vi "PLC.Dial750.vi"(7 "PLC Indicator":refnum<vi>, 8 "Is Child":bool, 9 "Config Dir":path=path "C:/MTE/Circle Test/Config", 10 "Name":string="PLC", 11 "TE Q":refnum<queue>) -> ()   [LabVIEW 2018]
uses:
  Controls/PLC.750 Variables.ctl
  <vilib>/KATE/Queues/Q.Element.ctl
  Controls/PLC750.Connection Config.ctl
  Controls/PLC750.Variable Names.ctl
  <vilib>/KATE/Queues/Queue Utils.lvlib
  <instrlib>/_Ackermann Automation/TwinCAT ADS Library/TcAdsLV_TCP/TcAdsLV_TCP_3.lvlib
  <vilib>/KATE/Scheduler/Scheduler.lvlib
  <vilib>/KATE/Time/Time Utils.lvlib
panel:
  out "Test State 2":T1(radio)
  out "Connected":bool
  in  "Tab Control":enum32{"Operate", "Config"}(tab)
  in  "Enabled":bool=TRUE
  in  "Clear Start":bool
  in  "Seq Done FAIL":bool
  in  "Clear Done":bool
  in  "Clear Pass":bool
  in  "Set Running":bool
  in  "Seq Run":bool
  in  "Seq Done PASS":bool
  in  "Seq Start Capture":bool
  out "Status":string
  out "Nest":string
  out "SN":string
  out "Test State":T1(radio)
  out "Reading":bool
  out "PLC Variables":T2
  in  "Set Ready":bool
  out "Test Running":bool
  out "Result":string="PASS"
  out "Read Time":timestamp format="%<%.3X>T"
  in  "PLC Read Interval(s)":dbl=0.1 caption="Read Interval(s)" format="%#_13g"
  in  "Read Data":bool
  in  "Clear Running":bool
  in  "Exit":bool
  in  "Clear Error":bool
  out "Error Time":timestamp format="%<%.3X>T"
  out "Connection Info":T3={"Net ID Target"="5.49.203.74.1.1", "Net ID Source"="192.168.1.18.1.1", "IP Address Target"="172.16.113.5", "Target Port"=851}
  out "Error":errorcluster
  in  "Retry Sec":dbl=2.0 caption="Connect Retry Sec" format="%#_13g"
  out "VarNames":T4={"SN"="g.SN", "Nest"="g.Nest", "Ready"="g.Ready", "Start"="g.Start", "Pass"="g.Pass", "Done"="g.Done", "Running"="GVL.gDone"}
  in  "Reset":bool
  in  "Single Step":bool
  in  "Emulate":bool
  out "Activation Ok":bool
  # "PLC Connection Manager"
  # "*** Sequence ***\nPLC -> \n  Set Done=F\n  Set Pass=F\n  Set Start=F\n  Set Running=F\n  Set Nest = Value\n  Set SN = Value\n  Set Ready=T\n\nTE -> \n  Get Nest\n  Get SN\n  Set Ready=F\n  Launch Test Sequence\n  \nTE -> \n  Test ready for tracked objects to spin\n   Set Start=T\n\nPLC -> \n  Set Running=T\n  Spin objects 360 deg\n  Set Running=F\n\nTE -> \n  Continue test\n  Test Complete\n   Set Pass = Value (T = Pass, F = Fail or Error)\n   Set Done=T\n\nPLC -> \n   Set Done=F"
  # "Simulate PLC"
  # "Test Executive Data"
  # "Simulate TE"
  # "Set Start"
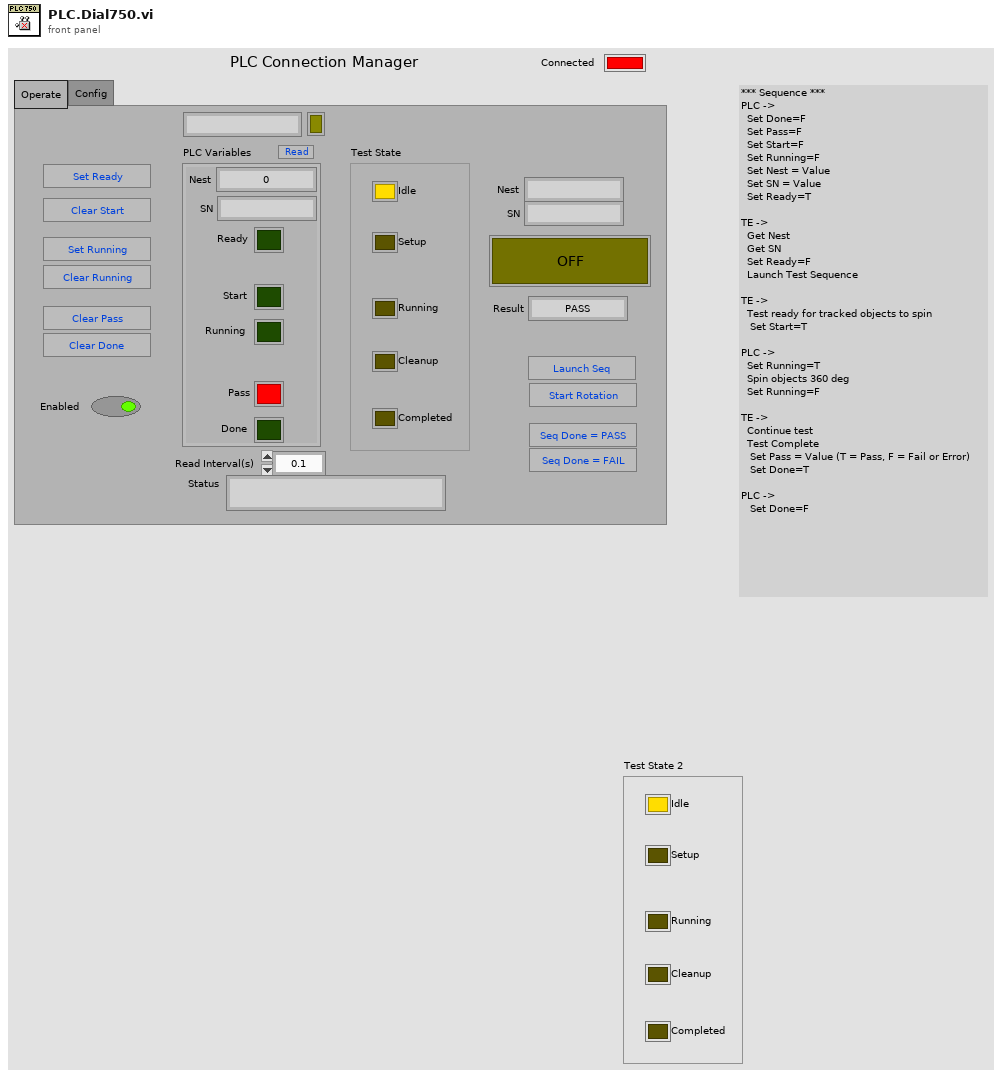
[diagram p1: front panel]
types:
  T1 = enum32{"Idle", "Setup", "Running", "Cleanup", "Completed"}
  T2 = typedef "PLC.750 Variables.ctl" = cluster{"Nest":i32, "SN":string, "Ready":bool, "Start":bool, "Pass":bool, "Done":bool, "Running":bool}
  T3 = typedef "PLC750.Connection Config.ctl" = cluster{"Net ID Target":string, "Net ID Source":string, "IP Address Target":string, "Target Port":u16}
  T4 = typedef "PLC750.Variable Names.ctl" = cluster{"SN":string, "Nest":string, "Ready":string, "Start":string, "Pass":string, "Done":string, "Running":string}
  T5 = enum8{"Enabled", "Disabled", "Disabled and Grayed Out"}
  T6 = enum32{"invalid app kind", "Development System", "Run Time System", "Student Edition", "Embedded LabVIEW", "Evaluation", "Custom"}
  T7 = enum32{"Invalid", "Standard", "Closed", "Hidden", "Minimized", "Maximized"}
  T8 = cluster{"VarConfig":T4, "Var Names":string[][], "Data":T2, "Session Ref":u32, "Connected":bool, "ConCfg":T3, "State":enum32{"Idle", "Setup", "Running", "Cleanup", "Completed"}, "PLC Indicator":refnum<vi>}
  T9 = typedef "TcAdsLV_Common_3.lvlib/ClusterAdsSymbolEntry.ctl" = cluster{"Index Group":u32, "Index Offset":u32, "Size":u32, "Data Type":u32, "Flags":u32, "Name":string, "Type":string, "Comment":string}
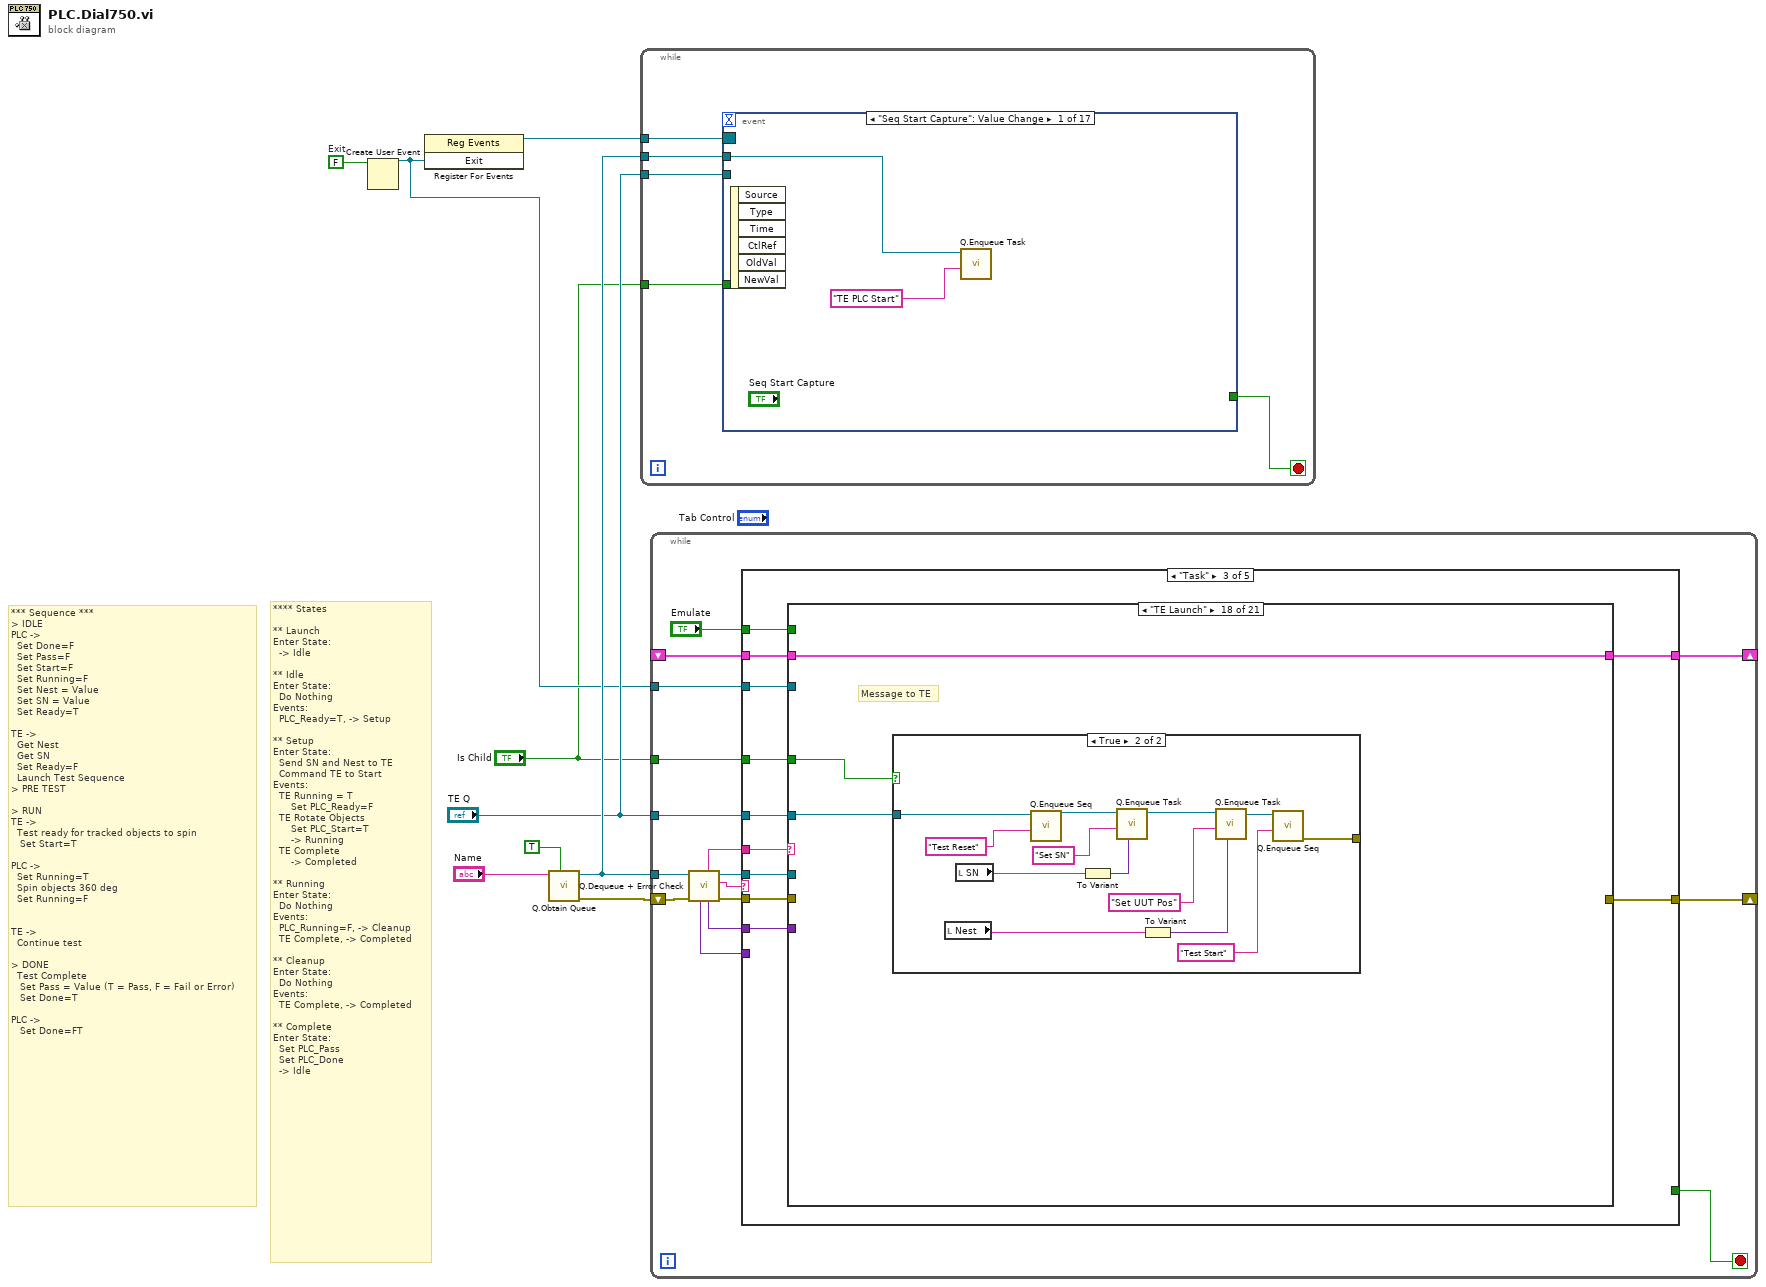
[diagram p0: block diagram]
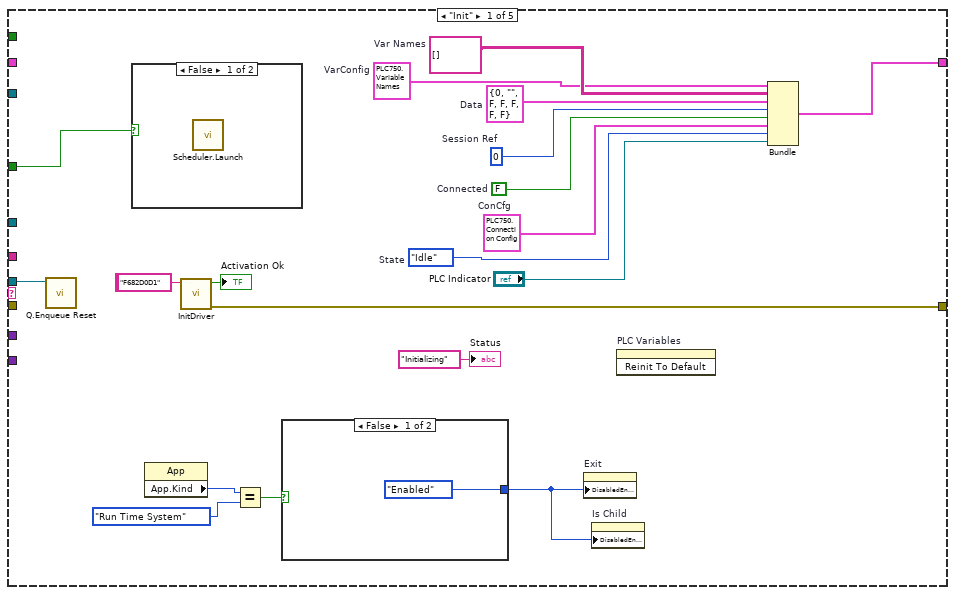
[diagram p2: hidden frame]
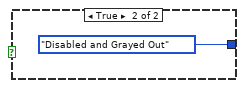
[diagram p3: hidden frame]
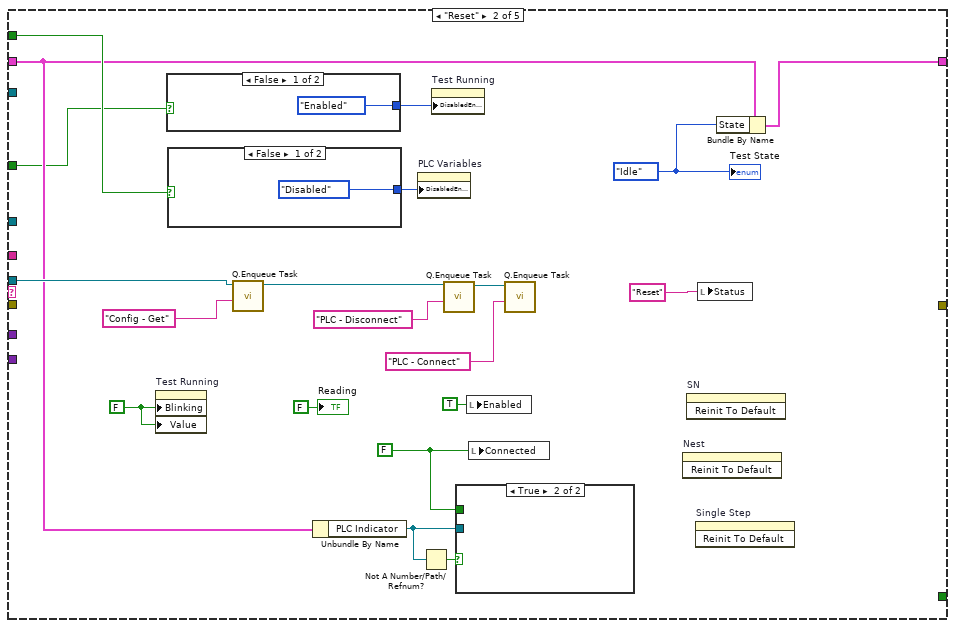
[diagram p5: hidden frame]
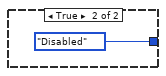
[diagram p6: hidden frame]
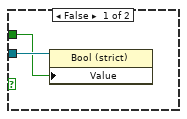
[diagram p7: hidden frame]
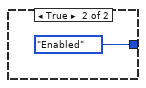
[diagram p8: hidden frame]
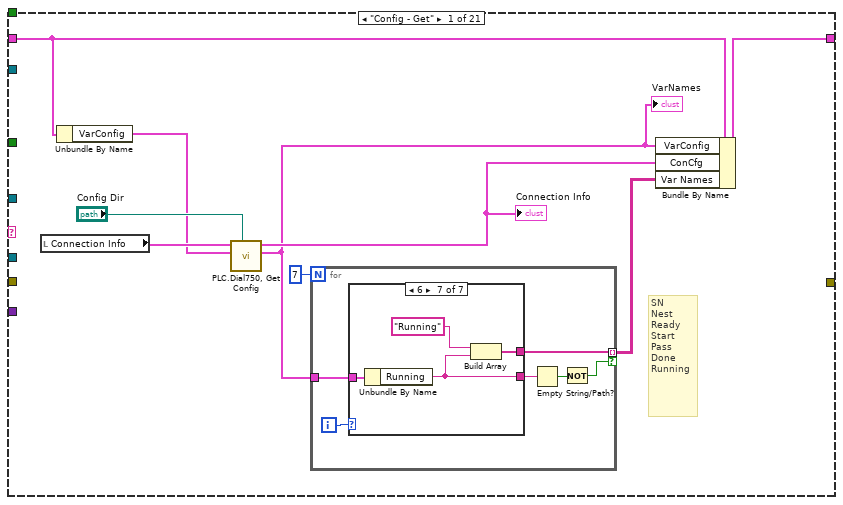
[diagram p9: hidden frame]
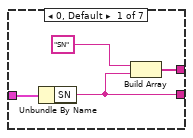
[diagram p10: hidden frame]
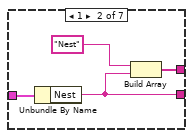
[diagram p11: hidden frame]
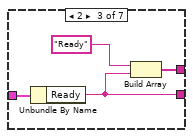
[diagram p12: hidden frame]
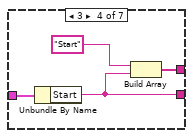
[diagram p13: hidden frame]
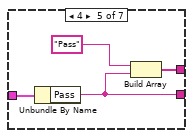
[diagram p14: hidden frame]
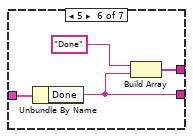
[diagram p15: hidden frame]
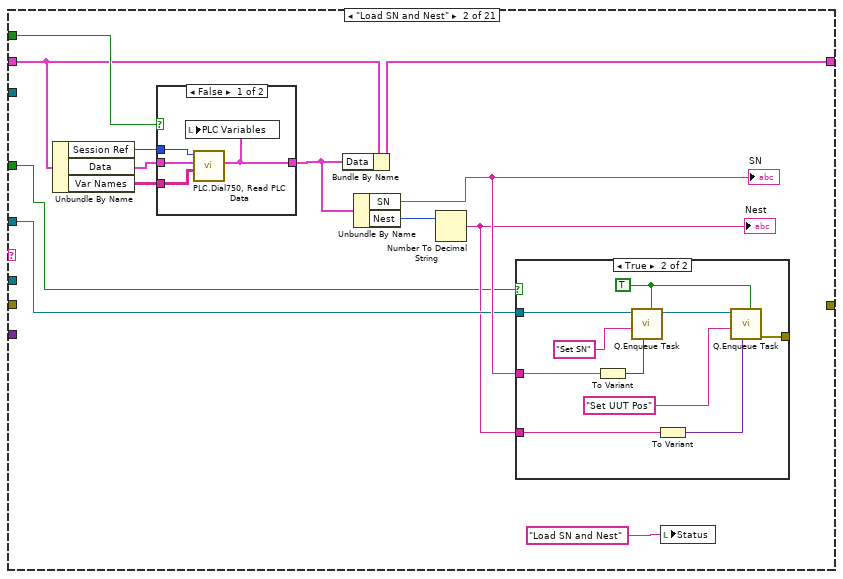
[diagram p16: hidden frame]
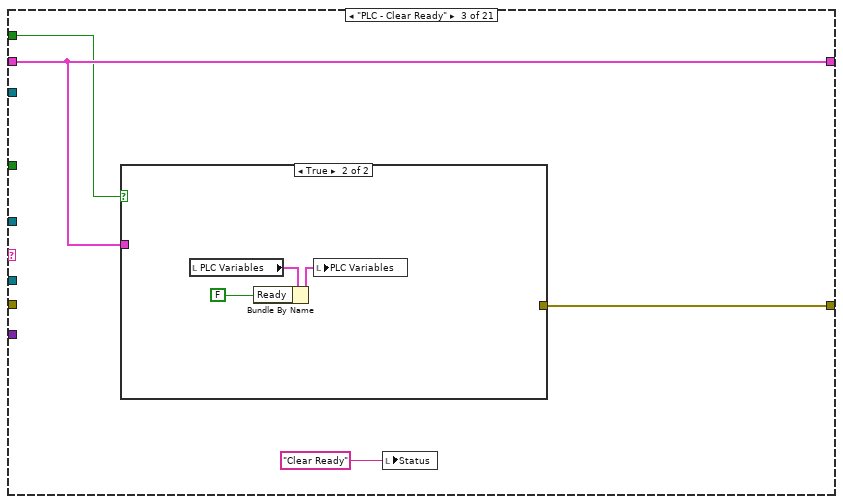
[diagram p19: hidden frame]
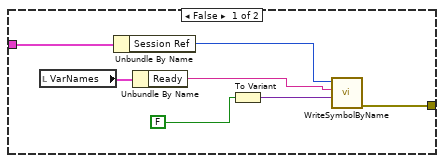
[diagram p20: hidden frame]
diagram:
  w6 = FALSE  # Exit
  # "**** States\n\n** Launch\nEnter State: \n  -> Idle\n\n** Idle\nEnter State: \n  Do Nothing\nEvents:\n  PLC_Ready=T, -> Setup\n\n** Setup\nEnter State: \n  Send SN and Nest to TE\n  Command TE to Start\nEvents:\n  TE Running = T\n      Set PLC_Ready=F\n  TE Rotate Objects\n      Set PLC_Start=T\n      -> Running\n  TE Complete\n      -> Completed\n\n** Running\nEnter State: \n  Do Nothing\nEvents:\n  PLC_Running=F, -> Cleanup\n  TE Complete, -> Completed\n\n** Cleanup\nEnter State: \n  Do Nothing\nEvents:\n  TE Complete, -> Completed\n\n** Complete\nEnter State: \n  Set PLC_Pass\n  Set PLC_Done \n  -> Idle"
  # "*** Sequence ***\n> IDLE\nPLC -> \n  Set Done=F\n  Set Pass=F\n  Set Start=F\n  Set Running=F\n  Set Nest = Value\n  Set SN = Value\n  Set Ready=T\n\nTE -> \n  Get Nest\n  Get SN\n  Set Ready=F\n  Launch Test Sequence\n> PRE TEST\n  \n> RUN\nTE -> \n  Test ready for tracked objects to spin\n   Set Start=T\n\nPLC -> \n  Set Running=T\n  Spin objects 360 deg\n  Set Running=F\n\n\nTE -> \n  Continue test\n\n> DONE\n  Test Complete\n   Set Pass = Value (T = Pass, F = Fail or Error)\n   Set Done=T\n\nPLC -> \n   Set Done=FT"
  n1 = Create User Event(user event datatype=w6) -> (user event=w2:refnum<user-event>)  [unwired: 1 in, 1 out]
  n2 = register-events(w2) -> (reference out=w5:refnum<event-registration>)  [unwired: 2 in, 1 out]
  n3 = call <vilib>:"Q.Obtain Queue.vi"("Enqueue Init"=TRUE, "Q Name"="Name") -> ("error out"=w3:errorcluster, "Q Out"=w7:refnum<queue>)  [unwired: 7 in, 1 out]
  n4 = while {
    tunnel: w7 -> [w14]
    tunnel: w5 -> [w13]
    tunnel: "TE Q" -> [w12]
    tunnel: "Is Child" -> [w10]
    stop <- w11 stop-if-true
    n5 = event shown="[0] \"Seq Start Capture\": Value Change" {
      selector: w13 -> [_ _ _ _ _ _ _ _ _ _ _ _ _ _ _ _ _]
      dyn-events: _ -> [_ _ _ _ _ _ _ _ _ _ _ _ _ _ _ _ _]
      timeout: _ -> [_ _ _ _ _ _ _ _ _ _ _ _ _ _ _ _ _]
      tunnel: w14 -> [w16 _ _ w21 w22 _ w32 w38 _ _ _ _ _ _ w57 w63 w64]
      tunnel: w12 -> [_ _ _ _ _ _ _ _ _ _ _ _ _ _ _ _ _]
      tunnel: [_ _ _ _ _ _ _ _ TRUE _ _ _ _ _ w56 TRUE _] -> w11
      tunnel: w10 -> [_ _ _ _ _ _ _ _ _ _ _ _ _ _ w55 _ _]
      event "Seq Start Capture": Value Change {
        n6 = event-data() -> ()  [unwired: 1 in, 6 out]
        n7 = call <vilib>:"Q.Enqueue Task.vi"("Task Name"="TE PLC Start", "Q In"=w16) -> ()  [unwired: 8 in, 2 out]
      }
      event "Emulate": Value Change {
        n8 = event-data() -> ("NewVal"=w17:bool)  [unwired: 1 in, 5 out]
        n9 = case shown="False" w17 {
          tunnel: [T5."Disabled" ("Disabled") T5."Enabled" ("Disabled")] -> w18
          frame False {
          }
          frame True {
          }
        }
        n10 = property on="PLC Variables" class="Clust (strict)"("DisabledEnum"=w18) -> ()  [unwired: 2 in, 2 out]
      }
      event "Clear Error": Value Change {
        n11 = event-data() -> ()  [unwired: 1 in, 6 out]
        n12 = invoke on="Error" class="Clust (strict)" method="Reinit To Default"() -> ()  [unwired: 3 in, 3 out]
      }
      event "Reset": Value Change {
        n13 = event-data() -> ()  [unwired: 1 in, 6 out]
        n14 = call <vilib>:"Q.Enqueue Reset.vi"("Q In"=w21) -> ()  [unwired: 9 in, 2 out]
      }
      event "Read Data": Value Change {
        n15 = event-data() -> ()  [unwired: 1 in, 6 out]
        n16 = call <vilib>:"Q.Enqueue Task.vi"("Task Name"="PLC - Read Data", "Q In"=w22) -> ()  [unwired: 8 in, 2 out]
      }
      event "Set Ready": Value Change {
        n17 = event-data() -> ()  [unwired: 1 in, 6 out]
        n18 = local read "PLC Variables"() -> (w25:T2)
        n19 = Bundle By Name(cluster=w25, "Ready"=TRUE) -> (w26:T2)
        n20 = local write "PLC Variables"(w26) -> ()
      }
      event "Seq Done PASS": Value Change {
        n21 = event-data() -> ()  [unwired: 1 in, 6 out]
        n22 = To Variant(anything="PASS") -> (Variant=w27:variant)
        n23 = call <vilib>:"Q.Enqueue Task.vi"("Data1"=w27, "Task Name"="TE Result", "Q In"=w32) -> ("Q Out"=w30:refnum<queue>)  [unwired: 7 in, 1 out]
        n24 = call <vilib>:"Q.Enqueue Task.vi"("Task Name"="TE Complete", "Q In"=w30) -> ()  [unwired: 8 in, 2 out]
      }
      event "Seq Done FAIL": Value Change {
        n25 = event-data() -> ()  [unwired: 1 in, 6 out]
        n26 = To Variant(anything="FAIL") -> (Variant=w33:variant)
        n27 = call <vilib>:"Q.Enqueue Task.vi"("Data1"=w33, "Task Name"="TE Result", "Q In"=w38) -> ("Q Out"=w36:refnum<queue>)  [unwired: 7 in, 1 out]
        n28 = call <vilib>:"Q.Enqueue Task.vi"("Task Name"="TE Complete", "Q In"=w36) -> ()  [unwired: 8 in, 2 out]
      }
      event User Event {
        n29 = event-data() -> ()  [unwired: 1 in, 4 out]
      }
      event "Set Running": Value Change {
        n30 = event-data() -> ()  [unwired: 1 in, 6 out]
        n31 = local read "PLC Variables"() -> (w40:T2)
        n32 = Bundle By Name(cluster=w40, "Running"=TRUE ("Ready")) -> (w41:T2)
        n33 = local write "PLC Variables"(w41) -> ()
      }
      event "Clear Done": Value Change {
        n34 = event-data() -> ()  [unwired: 1 in, 6 out]
        n35 = local read "PLC Variables"() -> (w43:T2)
        n36 = Bundle By Name(cluster=w43, "Done"=FALSE ("Ready")) -> (w44:T2)
        n37 = local write "PLC Variables"(w44) -> ()
      }
      event "Clear Start": Value Change {
        n38 = event-data() -> ()  [unwired: 1 in, 6 out]
        n39 = local read "PLC Variables"() -> (w46:T2)
        n40 = Bundle By Name(cluster=w46, "Start"=FALSE ("Ready")) -> (w47:T2)
        n41 = local write "PLC Variables"(w47) -> ()
      }
      event "Clear Pass": Value Change {
        n42 = event-data() -> ()  [unwired: 1 in, 6 out]
        n43 = local read "PLC Variables"() -> (w49:T2)
        n44 = Bundle By Name(cluster=w49, "Pass"=FALSE ("Ready")) -> (w50:T2)
        n45 = local write "PLC Variables"(w50) -> ()
      }
      event "Clear Running": Value Change {
        n46 = event-data() -> ()  [unwired: 1 in, 6 out]
        n47 = local read "PLC Variables"() -> (w52:T2)
        n48 = Bundle By Name(cluster=w52, "Running"=FALSE ("Ready")) -> (w53:T2)
        n49 = local write "PLC Variables"(w53) -> ()
      }
      event Panel Close? {
        n50 = event-data() -> ()  [unwired: 1 in, 4 out]
        n51 = case shown="False" w55 {
          tunnel: w57 -> [w60 _]
          tunnel: [TRUE _] -> w56
          frame False {
            n52 = call <vilib>:"Q.Enqueue Exit.vi"("Q In"=w60) -> ()  [unwired: 9 in, 2 out]
          }
          frame True {
            n53 = control-ref of="This VI"() -> (w61:refnum<vi>)
            n54 = invoke class="VI" method="FP.Close"(reference=w61) -> ()  [unwired: 2 in, 3 out]
          }
        }
        n55 = event-data("Discard?"=TRUE) -> ()  [unwired: 1 in, 1 out]
      }
      event "Exit": Value Change {
        n56 = event-data() -> ()  [unwired: 1 in, 6 out]
        n57 = call <vilib>:"Q.Enqueue Exit.vi"("Q In"=w63) -> ()  [unwired: 9 in, 2 out]
      }
      event "Seq Run": Value Change {
        n58 = event-data() -> ()  [unwired: 1 in, 6 out]
        n59 = call <vilib>:"Q.Enqueue Task.vi"("Task Name"="TE Running", "Q In"=w64) -> ()  [unwired: 8 in, 2 out]
      }
    }
  }
  n60 = while {
    tunnel: w7 -> [w81]
    shift-right: [w73] -> _
    shift-left: _ -> [w80]
    tunnel: "TE Q" -> [w71]
    shift-right: [w69] -> _
    shift-left: w3 -> [w70]
    tunnel: w2 -> [w68]
    tunnel: "Is Child" -> [w66]
    stop <- w72 stop-if-true
    n61 = call <vilib>:"Q.Dequeue + Error Check.vi"("Error In"=w70, "Q In"=w81) -> ("error out"=w77:errorcluster, "Cmd"=w79:string, "Q Out"=w78:refnum<queue>, "Data1"=w75:variant, "Sub"=w76:string, "Data2"=w74:variant)  [unwired: 4 in]
    n62 = case shown="\"Task\"" w79 {
      tunnel: w80 -> [_ w106 w135 w481 w495]
      tunnel: w78 -> [w93 w116 w137 _ _]
      tunnel: w77 -> [_ _ w136 w484 _]
      tunnel: w76 -> [_ _ w139 w485 _]
      tunnel: w75 -> [_ _ w138 w482 _]
      tunnel: w74 -> [_ _ _ _ _]
      tunnel: [w100 w117 w134 w481 w495] -> w73
      tunnel: [_ _ _ _ TRUE] -> w72
      tunnel: w71 -> [_ _ w130 _ _]
      tunnel: [w97 _ w133 _ _] -> w69
      tunnel: w68 -> [_ _ w132 _ w494]
      tunnel: "Emulate" -> [_ w112 w131 _ _]
      tunnel: w66 -> [w87 w104 w129 _ w492]
      frame "Init" {
        w90 = T1."Idle"  # State
        w91 = T4 {"SN"="g.SN", "Nest"="g.Nest", "Ready"="g.Ready", "Start"="", "Pass"="g.Pass", "Done"="g.Done", "Running"=""}  # VarConfig
        w92 = string[][] []  # Var Names
        w94 = T3 {"Net ID Target"="5.49.203.74.1.1", "Net ID Source"="192.168.1.18.1.1", "IP Address Target"="172.16.113.5", "Target Port"=851}  # ConCfg
        w95 = FALSE  # Connected
        w96 = u32 0  # Session Ref
        (unwired) "" ("License Number")
        w99 = T2 {"Nest"=0, "SN"="", "Ready"=FALSE, "Start"=FALSE, "Pass"=FALSE, "Done"=FALSE, "Running"=FALSE}  # Data
        n63 = call <vilib>:"Q.Enqueue Reset.vi"("Q In"=w93) -> ()  [unwired: 9 in, 2 out]
        n64 = case shown="False" w87 {
          frame False {
            n65 = call <vilib>:"Scheduler.Launch.vi"() -> ()  [unwired: 9 in, 3 out]
          }
          frame True {
          }
        }
        n66 = property class="App"() -> ("App.Kind"=w85:T6)  [unwired: 2 in, 2 out]
        n67 = call <instrlib>:"InitDriver.vi"("License Number"="F682D0D1") -> ("error out"=w97:errorcluster, "Activation Ok"=→"Activation Ok":bool)  [unwired: 8 in, 1 out]
        n68 = Equal?(x=w85, y=T6."Run Time System" ("Application:Kind")) -> (x = y?=w83:bool)
        n69 = case shown="False" w83 {
          tunnel: [T5."Enabled" ("Disabled") T5."Disabled and Grayed Out" ("Disabled")] -> w86
          frame False {
          }
          frame True {
          }
        }
        n70 = property on="Exit" class="Bool"("DisabledEnum"=w86) -> ()  [unwired: 2 in, 2 out]
        n71 = property on="Is Child" class="Bool (strict)"("DisabledEnum"=w86) -> ()  [unwired: 2 in, 2 out]
        n72 = invoke on="PLC Variables" class="Clust (strict)" method="Reinit To Default"() -> ()  [unwired: 3 in, 3 out]
        n73 = Bundle("VarConfig"=w91, "Var Names"=w92, "Data"=w99, "Session Ref"=w96, "Connected"=w95, "ConCfg"=w94, "State"=w90, "PLC Indicator"="PLC Indicator") -> (w100:T8)  [unwired: 1 in]
        "Status" <- "Initializing" ("Activity")
      }
      frame "Reset" {
        w113 = T1."Idle" ("Test State")
        w107 = FALSE ("Connected")
        w115 = FALSE ("Blinking")
        n74 = property on="Test Running" class="Bool (strict)"("Blinking"=w115, "Value"=w115) -> ()  [unwired: 2 in, 2 out]
        n75 = case shown="False" w104 {
          tunnel: [T5."Enabled" ("Disabled") T5."Disabled" ("Disabled")] -> w105
          frame False {
          }
          frame True {
          }
        }
        n76 = case shown="False" w112 {
          tunnel: [T5."Disabled" ("Disabled") T5."Enabled" ("Disabled")] -> w111
          frame False {
          }
          frame True {
          }
        }
        n77 = call <vilib>:"Q.Enqueue Task.vi"("Task Name"="Config - Get", "Q In"=w116) -> ("Q Out"=w118:refnum<queue>)  [unwired: 8 in, 1 out]
        n78 = Unbundle By Name(w106) -> ("PLC Indicator"=w108:refnum<vi>)
        n79 = property on="PLC Variables" class="Clust (strict)"("DisabledEnum"=w111) -> ()  [unwired: 2 in, 2 out]
        n80 = Not A Number/Path/Refnum?(number/path/refnum=w108) -> (NaN/Path/Refnum?=w109:bool)
        n81 = property on="Test Running" class="Bool (strict)"("DisabledEnum"=w105) -> ()  [unwired: 2 in, 2 out]
        n82 = call <vilib>:"Q.Enqueue Task.vi"("Task Name"="PLC - Disconnect", "Q In"=w118) -> ("Q Out"=w121:refnum<queue>)  [unwired: 8 in, 1 out]
        n83 = case shown="True" w109 {
          tunnel: w108 -> [w126 _]
          tunnel: w107 -> [w125 _]
          frame False {
            n84 = property class="Bool (strict)"(reference=w126, "Value"=w125) -> ()  [unwired: 1 in, 2 out]
          }
          frame True {
          }
        }
        n85 = local write "Enabled"(TRUE ("Enabled")) -> ()
        n86 = local write "Connected"(w107) -> ()
        n87 = call <vilib>:"Q.Enqueue Task.vi"("Task Name"="PLC - Connect", "Q In"=w121) -> ()  [unwired: 8 in, 2 out]
        n88 = invoke on="Nest" class="Str" method="Reinit To Default"() -> ()  [unwired: 3 in, 3 out]
        n89 = invoke on="SN" class="Str" method="Reinit To Default"() -> ()  [unwired: 3 in, 3 out]
        n90 = invoke on="Single Step" class="Bool (strict)" method="Reinit To Default"() -> ()  [unwired: 3 in, 3 out]
        n91 = local write "Status"("Reset" ("Activity")) -> ()
        n92 = Bundle By Name(cluster=w106, "State"=w113) -> (w117:T8)
        "Reading" <- FALSE ("Reading")
        "Test State" <- w113
      }
      frame "Task" {
        n93 = case shown="\"TE Launch\"" w139 {
          tunnel: w138 -> [_ _ _ _ _ _ _ _ _ _ _ _ _ _ w446 _ _ _ w472 _ _]
          tunnel: w137 -> [_ _ _ w233 _ w293 _ _ _ _ w373 w380 _ w438 _ _ w450 _ w469 w475 _]
          tunnel: w136 -> [_ _ _ _ _ w285 _ _ _ _ _ _ _ _ _ _ _ _ _ _ _]
          tunnel: w135 -> [w142 w183 w213 w229 w270 w292 w318 w334 w351 w365 w372 w379 w437 w442 w447 w448 w449 w454 w473 w478 w479]
          tunnel: [w147 w186 w213 w234 w270 w291 w318 w334 w351 w365 w371 w378 w437 w441 w447 w448 w449 w454 w473 w478 w479] -> w134
          tunnel: [_ _ w214 w232 _ w286 w319 w337 w352 _ _ _ _ _ _ _ _ _ _ _ _] -> w133
          tunnel: w132 -> [_ _ _ _ _ _ _ _ _ _ _ _ _ _ _ _ _ _ _ _ _]
          tunnel: w131 -> [_ w184 w212 w230 w273 w281 w316 w333 w350 _ _ _ _ _ _ _ _ _ _ _ _]
          tunnel: w130 -> [_ w192 _ _ _ _ _ _ _ _ _ w377 _ _ _ _ _ w453 _ _ _]
          tunnel: w129 -> [_ w190 _ _ _ _ _ _ _ _ _ _ _ _ _ _ _ w452 _ _ _]
          frame "Config - Get" {
            # "SN\nNest\nReady\nStart\nPass\nDone\nRunning"
            n94 = local read "Connection Info"() -> (w145:T3)
            n95 = Unbundle By Name(w142) -> ("VarConfig"=w141:T4)
            n96 = call "PLC.Dial750, Get Config.vi"("Config Folder"="Config Dir", "VarNames In"=w141, "Connection Info In"=w145) -> ("VarNames"=w143:T4, "Connection Info"=w146:T3)  [unwired: 6 in, 1 out]
            "VarNames" <- w143
            "Connection Info" <- w146
            n97 = for {
              N: 7 -> [_]
              tunnel: w143 -> [w154]
              tunnel: [w152] -> w144 mode=indexing if=w150
              i -> [w153]
              n98 = case shown="6" w153 {
                tunnel: w154 -> [w158 w162 w166 w170 w174 w178 w182]
                tunnel: [w156 w160 w164 w168 w172 w176 w180] -> w152
                tunnel: [w155 w159 w163 w167 w171 w175 w179] -> w149
                frame 0, Default {
                  n99 = Unbundle By Name(w158) -> ("SN"=w155:string)
                  n100 = Build Array("SN", w155) -> (w156:string[])
                }
                frame 1 {
                  n101 = Unbundle By Name(w162) -> ("Nest"=w159:string)
                  n102 = Build Array("Nest", w159) -> (w160:string[])
                }
                frame 2 {
                  n103 = Unbundle By Name(w166) -> ("Ready"=w163:string)
                  n104 = Build Array("Ready", w163) -> (w164:string[])
                }
                frame 3 {
                  n105 = Unbundle By Name(w170) -> ("Start"=w167:string)
                  n106 = Build Array("Start", w167) -> (w168:string[])
                }
                frame 4 {
                  n107 = Unbundle By Name(w174) -> ("Pass"=w171:string)
                  n108 = Build Array("Pass", w171) -> (w172:string[])
                }
                frame 5 {
                  n109 = Unbundle By Name(w178) -> ("Done"=w175:string)
                  n110 = Build Array("Done", w175) -> (w176:string[])
                }
                frame 6 {
                  n111 = Unbundle By Name(w182) -> ("Running"=w179:string)
                  n112 = Build Array("Running", w179) -> (w180:string[])
                }
              }
              n113 = Empty String/Path?(string/path=w149) -> (empty?=w151:bool)
              n114 = Not(x=w151) -> (.not. x?=w150:bool)
            }
            n115 = Bundle By Name(cluster=w142, "VarConfig"=w143, "ConCfg"=w146, "Var Names"=w144) -> (w147:T8)
          }
          frame "Load SN and Nest" {
            n116 = Unbundle By Name(w183) -> ("Session Ref"=w187:u32, "Data"=w188:T2, "Var Names"=w189:string[][])
            n117 = case shown="False" w184 {
              tunnel: w187 -> [w199 _]
              tunnel: w188 -> [w198 w200]
              tunnel: w189 -> [w197 _]
              tunnel: [w196 w200] -> w185
              frame False {
                n118 = call "PLC.Dial750, Read PLC Data.vi"("Var Names"=w197, "PLC Vars In"=w198, "Session Ref"=w199) -> ("PLC Variables"=w196:T2)  [unwired: 6 in, 2 out]
                n119 = local write "PLC Variables"(w196) -> ()
              }
              frame True {
              }
            }
            n120 = Bundle By Name(cluster=w183, "Data"=w185) -> (w186:T8)
            n121 = Unbundle By Name(w185) -> ("SN"=w193:string, "Nest"=w195:i32)
            "SN" <- w193
            n122 = Number To Decimal String(number=w195) -> (decimal integer string=w191:string)  [unwired: 1 in]
            "Nest" <- w191
            n123 = case shown="True" w190 {
              tunnel: w193 -> [_ w210]
              tunnel: w192 -> [_ w209]
              tunnel: w191 -> [_ w208]
              tunnel: [_ w202] -> _
              frame False {
              }
              frame True {
                w201 = TRUE ("Top of Q")
                n124 = To Variant(anything=w210) -> (Variant=w207:variant)
                n125 = call <vilib>:"Q.Enqueue Task.vi"("Top of Q"=w201, "Data1"=w207, "Task Name"="Set SN", "Q In"=w209) -> ("Q Out"=w203:refnum<queue>)  [unwired: 6 in, 1 out]
                n126 = To Variant(anything=w208) -> (Variant=w205:variant)
                n127 = call <vilib>:"Q.Enqueue Task.vi"("Top of Q"=w201, "Data1"=w205, "Task Name"="Set UUT Pos", "Q In"=w203) -> ("error out"=w202:errorcluster)  [unwired: 6 in, 1 out]
              }
            }
            n128 = local write "Status"("Load SN and Nest" ("Activity")) -> ()
          }
          frame "PLC - Clear Ready" {
            n129 = case shown="True" w212 {
              tunnel: [w220 _] -> w214
              tunnel: w213 -> [w215 _]
              frame False {
                n130 = local read "VarNames"() -> (w221:T4)
                n131 = Unbundle By Name(w215) -> ("Session Ref"=w219:u32)
                n132 = Unbundle By Name(w221) -> ("Ready"=w218:string)
                n133 = To Variant(anything=FALSE) -> (Variant=w217:variant)
                n134 = call <instrlib>:"WriteSymbolByName.vi"("Data"=w217, "Name"=w218, "Session Ref"=w219) -> ("error out"=w220:errorcluster)  [unwired: 7 in, 1 out]
              }
              frame True {
                n135 = local read "PLC Variables"() -> (w223:T2)
                n136 = Bundle By Name(cluster=w223, "Ready"=FALSE) -> (w222:T2)
                n137 = local write "PLC Variables"(w222) -> ()
              }
            }
            n138 = local write "Status"("Clear Ready" ("Activity")) -> ()
          }
          frame "PLC - Connect" {
            n139 = Unbundle By Name(w229) -> ("ConCfg"=w231:T3)
            n140 = case shown="False" w230 {
              tunnel: [w242 _] -> w235
              tunnel: w231 -> [w241 _]
              tunnel: [w239 _] -> w225
              tunnel: [w238 _] -> _
              frame False {
                n141 = Unbundle By Name(w241) -> ("Net ID Source"=w247:string, "IP Address Target"=w246:string, "Net ID Target"=w245:string, "Target Port"=w244:u16)
                n142 = call <instrlib>:"OpenAdsSession.vi"("Net ID Source"=w247, "Query Symbols"=TRUE, "IP Address Target"=w246, "timeout ms"=2000, "Target Port"=w244, "Net ID Target"=w245) -> ("error out"=w242:errorcluster, "Symbols"=w238:T9[], "Session Ref"=w239:u32)  [unwired: 1 in, 2 out]
              }
              frame True {
                n143 = Wait (ms)(milliseconds to wait=u32 100) -> ()  [unwired: 1 out]
              }
            }
            n144 = case shown="Error" w235 {
              selector: w235 -> [_ w262]
              tunnel: [w256 w264] -> w234
              tunnel: w229 -> [w255 w265]
              tunnel: w233 -> [w252 w261]
              tunnel: [TRUE _] -> w226
              tunnel: [_ w262] -> w232
              tunnel: w225 -> [w250 w258]
              frame No Error {
                n145 = Get Date/Time In Seconds() -> (seconds since 1Jan1904=w249:timestamp)
                n146 = local write "Read Time"(w249) -> ()
                n147 = call <vilib>:"Q.Enqueue Task.vi"("Task Name"="PLC - Read Data" ("Sched Name"), "Q In"=w252) -> ()  [unwired: 8 in, 2 out]
                n148 = Bundle By Name(cluster=w255, "Connected"=TRUE, "Session Ref"=w250) -> (w256:T8)
              }
              frame Error {
                n149 = call <instrlib>:"CloseAdsSession.vi"("Session Ref"=w258) -> ("error out"=w257:errorcluster)  [unwired: 10 in]
                n150 = local read "Single Step"() -> (w260:bool)
                n151 = case shown="False" w260 {
                  tunnel: w261 -> [w266 _]
                  frame False {
                    w268 = "PLC - Connect" ("Sched Name")
                    n152 = call <vilib>:"Scheduler.AddTask.vi"("Interval(s)"="Retry Sec", "Task Name"=w268, "Sched Name"=w268, "Q In"=w266) -> ()  [unwired: 6 in, 2 out]
                  }
                  frame True {
                  }
                }
                n153 = call <vilib>:"Clear Errors.vi"("error in (no error)"=w257) -> ()  [unwired: 5 in, 2 out]
                n154 = Get Date/Time In Seconds() -> (seconds since 1Jan1904=w259:timestamp)
                n155 = local write "Read Time"(w259) -> ()
                n156 = Bundle By Name(cluster=w265, "Connected"=FALSE) -> (w264:T8)
              }
            }
            "Connected" <- w226
            n157 = Unbundle By Name(w229) -> ("PLC Indicator"=w227:refnum<vi>)
            n158 = Not A Number/Path/Refnum?(number/path/refnum=w227) -> (NaN/Path/Refnum?=w228:bool)
            n159 = case shown="True" w228 {
              tunnel: w227 -> [w237 _]
              tunnel: w226 -> [w236 _]
              frame False {
                n160 = property class="Bool (strict)"(reference=w237, "Value"=w236) -> ()  [unwired: 1 in, 2 out]
              }
              frame True {
              }
            }
          }
          frame "PLC - Disconnect" {
            w269 = FALSE ("Connected")
            n161 = case shown="False" w273 {
              tunnel: w270 -> [w277 _]
              frame False {
                n162 = Unbundle By Name(w277) -> ("Session Ref"=w276:u32)
                n163 = call <instrlib>:"CloseAdsSession.vi"("Session Ref"=w276) -> ("error out"=w278:errorcluster)  [unwired: 10 in]
                n164 = call <vilib>:"Clear Errors.vi"("error in (no error)"=w278) -> ()  [unwired: 5 in, 2 out]
              }
              frame True {
              }
            }
            n165 = Unbundle By Name(w270) -> ("PLC Indicator"=w271:refnum<vi>)
            n166 = Not A Number/Path/Refnum?(number/path/refnum=w271) -> (NaN/Path/Refnum?=w272:bool)
            n167 = case shown="False" w272 {
              tunnel: w271 -> [w275 _]
              tunnel: w269 -> [w274 _]
              frame False {
                n168 = property class="Bool (strict)"(reference=w275, "Value"=w274) -> ()  [unwired: 1 in, 2 out]
              }
              frame True {
              }
            }
            n169 = local write "Connected"(w269) -> ()
          }
          frame "PLC - Read Data" {
            n170 = flat-sequence {
              tunnel: w285 -> [w302]
              tunnel: [w302] -> w284
              frame #0 {
                n171 = local write "Reading"(TRUE ("Reading")) -> ()
              }
            }
            n172 = Unbundle By Name(w292) -> ("Session Ref"=w290:u32, "Data"=w289:T2, "Var Names"=w288:string[][])
            n173 = Get Date/Time In Seconds() -> (seconds since 1Jan1904=→"Read Time":timestamp)
            n174 = case shown="False" w281 {
              tunnel: w290 -> [w299 _]
              tunnel: w289 -> [w298 _]
              tunnel: w288 -> [w297 _]
              tunnel: [w296 _] -> w287
              tunnel: w284 -> [w295 _]
              tunnel: [w294 w300] -> w279
              frame False {
                n175 = call "PLC.Dial750, Read PLC Data.vi"("error in (no error)"=w295, "Var Names"=w297, "PLC Vars In"=w298, "Session Ref"=w299) -> ("error out"=w296:errorcluster, "PLC Variables"=w294:T2)  [unwired: 5 in, 1 out]
                "PLC Variables" <- w294
              }
              frame True {
                n176 = local read "PLC Variables"() -> (w300:T2)
                n177 = Wait (ms)(milliseconds to wait=u32 100) -> ()  [unwired: 1 out]
              }
            }
            n178 = local write "Status"("Read" ("Activity")) -> ()
            n179 = Bundle By Name(cluster=w292, "Data"=w279) -> (w291:T8)
            n180 = case shown="No Error" w287 {
              selector: w287 -> [_ w312]
              tunnel: w293 -> [w307 w313]
              tunnel: [_ w312] -> w286
              tunnel: [FALSE ("Reading") _] -> w283
              frame No Error {
                n181 = call <vilib>:"Q.Enqueue Task.vi"("Task Name"="State Check", "Q In"=w307) -> ("Q Out"=w306:refnum<queue>)  [unwired: 8 in, 1 out]
                n182 = case shown="False" "Single Step" {
                  tunnel: w306 -> [w310 _]
                  frame False {
                    w311 = "PLC - Read Data" ("Sched Name")
                    n183 = call <vilib>:"Scheduler.AddTask.vi"("Interval(s)"="PLC Read Interval(s)", "Task Name"=w311, "Sched Name"=w311, "Q In"=w310) -> ()  [unwired: 6 in, 2 out]
                  }
                  frame True {
                  }
                }
              }
              frame Error {
                w315 = "PLC - Connect" ("Sched Name")
                n184 = call <vilib>:"Scheduler.AddTask.vi"("Interval(s)"=1.0, "Task Name"=w315, "Sched Name"=w315, "Q In"=w313) -> ()  [unwired: 6 in, 2 out]
              }
            }
            n185 = local write "Reading"(w283) -> ()
          }
          frame "PLC - Set Done" {
            n186 = case shown="True" w316 {
              tunnel: [w325 _] -> w319
              tunnel: w318 -> [w320 _]
              frame False {
                n187 = local read "VarNames"() -> (w326:T4)
                n188 = Unbundle By Name(w320) -> ("Session Ref"=w324:u32)
                n189 = Unbundle By Name(w326) -> ("Done"=w323:string)
                n190 = To Variant(anything=TRUE) -> (Variant=w322:variant)
                n191 = call <instrlib>:"WriteSymbolByName.vi"("Data"=w322, "Name"=w323, "Session Ref"=w324) -> ("error out"=w325:errorcluster)  [unwired: 7 in, 1 out]
              }
              frame True {
                n192 = local read "PLC Variables"() -> (w328:T2)
                n193 = Bundle By Name(cluster=w328, "Done"=TRUE ("Ready")) -> (w329:T2)
                n194 = Wait (ms)(milliseconds to wait=u32 100) -> ()  [unwired: 1 out]
                n195 = local write "PLC Variables"(w329) -> ()
              }
            }
            n196 = local write "Status"("Set Done" ("Activity")) -> ()
          }
          frame "PLC - Set Result" {
            n197 = local read "Result"() -> (w331:string)
            n198 = Equal?(x=w331, y="PASS") -> (x = y?=w335:bool)
            n199 = case shown="True" w333 {
              tunnel: [w343 _] -> w337
              tunnel: w335 -> [w339 w345]
              tunnel: w334 -> [w338 _]
              frame False {
                n200 = local read "VarNames"() -> (w344:T4)
                n201 = Unbundle By Name(w338) -> ("Session Ref"=w342:u32)
                n202 = To Variant(anything=w339) -> (Variant=w340:variant)
                n203 = Unbundle By Name(w344) -> ("Pass"=w341:string)
                n204 = call <instrlib>:"WriteSymbolByName.vi"("Data"=w340, "Name"=w341, "Session Ref"=w342) -> ("error out"=w343:errorcluster)  [unwired: 7 in, 1 out]
              }
              frame True {
                n205 = local read "PLC Variables"() -> (w346:T2)
                n206 = Bundle By Name(cluster=w346, "Pass"=w345) -> (w347:T2)
                n207 = Wait (ms)(milliseconds to wait=u32 100) -> ()  [unwired: 1 out]
                n208 = local write "PLC Variables"(w347) -> ()
              }
            }
            n209 = local write "Status"("Set Result" ("Activity")) -> ()
          }
          frame "PLC - Set Start" {
            n210 = case shown="False" w350 {
              tunnel: [w358 _] -> w352
              tunnel: w351 -> [w353 _]
              frame False {
                n211 = local read "VarNames"() -> (w359:T4)
                n212 = Unbundle By Name(w353) -> ("Session Ref"=w357:u32)
                n213 = Unbundle By Name(w359) -> ("Start"=w356:string)
                n214 = To Variant(anything=TRUE) -> (Variant=w355:variant)
                n215 = call <instrlib>:"WriteSymbolByName.vi"("Data"=w355, "Name"=w356, "Session Ref"=w357) -> ("error out"=w358:errorcluster)  [unwired: 7 in, 1 out]
              }
              frame True {
                n216 = local read "PLC Variables"() -> (w360:T2)
                n217 = Bundle By Name(cluster=w360, "Start"=TRUE ("Ready")) -> (w361:T2)
                n218 = local write "PLC Variables"(w361) -> ()
              }
            }
            n219 = local write "Status"("Set Start" ("Activity")) -> ()
          }
          frame "Sim - Clear Done" {
            n220 = call <vilib>:"Time.Inline Delay.vi"("Wait(secs)"=1.0) -> ("error out"=w364:errorcluster)  [unwired: 9 in, 1 out]
            n221 = flat-sequence {
              tunnel: w364 -> [_]
              frame #0 {
                w366 = FALSE ("Ready")
                n222 = local read "PLC Variables"() -> (w367:T2)
                n223 = Bundle By Name(cluster=w367, "Done"=w366, "Pass"=w366) -> (w368:T2)
                n224 = local write "PLC Variables"(w368) -> ()
              }
            }
          }
          frame "Sim - Test Complete" {
            w369 = FALSE ("Blinking")
            w370 = T1."Completed" ("Test State")
            n225 = call <vilib>:"Q.Enqueue Task.vi"("Task Name"="PLC - Set Result", "Q In"=w373) -> ("Q Out"=w375:refnum<queue>)  [unwired: 8 in, 1 out]
            n226 = property on="Test Running" class="Bool (strict)"("Blinking"=w369, "Value"=w369) -> ()  [unwired: 2 in, 2 out]
            n227 = call <vilib>:"Q.Enqueue Task.vi"("Task Name"="PLC - Set Done", "Q In"=w375) -> ()  [unwired: 8 in, 2 out]
            n228 = Bundle By Name(cluster=w372, "State"=w370) -> (w371:T8)
            n229 = local write "Test State"(w370) -> ()
          }
          frame "State Check" {
            n230 = Unbundle By Name(w379) -> ("Data"=w381:T2, "State"=w382:T1)
            n231 = case shown="\"Setup\"" w382 {
              tunnel: w381 -> [_ w390 w403 w414 _ w425]
              tunnel: w380 -> [_ w389 _ _ _ _]
              tunnel: w379 -> [w383 w388 w405 w416 w423 w427]
              tunnel: [w383 w387 w404 w415 w423 w426] -> w378
              tunnel: w377 -> [_ _ w401 w412 _ _]
              frame Default {
                # "Do Nothing"
              }
              frame "Idle" {
                n232 = Unbundle By Name(w390) -> ("Ready"=w384:bool)
                n233 = And(x="Enabled", y=w384) -> (x .and. y?=w386:bool)
                n234 = case shown="True" w386 {
                  tunnel: w389 -> [_ w396]
                  tunnel: w388 -> [w391 w400]
                  tunnel: [w391 w399] -> w387
                  frame False {
                    # "Do Nothing"
                  }
                  frame True {
                    w398 = T1."Setup" ("Test State")
                    n235 = Wait (ms)(milliseconds to wait=u32 100) -> ()  [unwired: 1 out]
                    n236 = call <vilib>:"Q.Enqueue Task.vi"("Top of Q"=TRUE, "Task Name"="Load SN and Nest", "Q In"=w396) -> ("Q Out"=w394:refnum<queue>)  [unwired: 7 in, 1 out]
                    n237 = local write "Test State"(w398) -> ()
                    n238 = call <vilib>:"Q.Enqueue Task.vi"("Task Name"="TE Launch", "Q In"=w394) -> ()  [unwired: 8 in, 2 out]
                    n239 = Bundle By Name(cluster=w400, "State"=w398) -> (w399:T8)
                  }
                }
              }
              frame "Setup" {
                n240 = Unbundle By Name(w403) -> ("Running"=w402:bool)
                n241 = case shown="True" w402 {
                  tunnel: w405 -> [w406 w411]
                  tunnel: [w406 w410] -> w404
                  tunnel: w401 -> [_ w408]
                  frame False {
                  }
                  frame True {
                    w409 = T1."Running" ("Test State")
                    n242 = local write "Test State"(w409) -> ()
                    n243 = call <vilib>:"Q.Enqueue Task.vi"("Task Name"="PLC - Running Start", "Q In"=w408) -> ()  [unwired: 8 in, 2 out]
                    n244 = Bundle By Name(cluster=w411, "State"=w409) -> (w410:T8)
                  }
                }
              }
              frame "Running" {
                n245 = Unbundle By Name(w414) -> ("Running"=w413:bool)
                n246 = case shown="False" w413 {
                  tunnel: w416 -> [w421 w422]
                  tunnel: [w420 w422] -> w415
                  tunnel: w412 -> [w417 _]
                  frame False {
                    w419 = T1."Cleanup" ("Test State")
                    n247 = local write "Test State"(w419) -> ()
                    n248 = Bundle By Name(cluster=w421, "State"=w419) -> (w420:T8)
                    n249 = call <vilib>:"Q.Enqueue Task.vi"("Task Name"="PLC - Running Done", "Q In"=w417) -> ()  [unwired: 8 in, 2 out]
                  }
                  frame True {
                  }
                }
              }
              frame "Cleanup" {
              }
              frame "Completed" {
                n250 = Unbundle By Name(w425) -> ("Done"=w424:bool)
                n251 = case shown="False" w424 {
                  tunnel: w427 -> [w430 w431]
                  tunnel: [w429 w431] -> w426
                  frame False {
                    w428 = T1."Idle" ("Test State")
                    n252 = local write "Test State"(w428) -> ()
                    n253 = Bundle By Name(cluster=w430, "State"=w428) -> (w429:T8)
                  }
                  frame True {
                  }
                }
              }
            }
          }
          frame "Show Panel" {
            n254 = control-ref of="This VI"() -> (w432:refnum<vi>)
            n255 = invoke class="VI" method="FP.Center"(reference=w432) -> (reference out=w435:refnum<vi>, error out=w436:errorcluster)  [unwired: 2 in, 1 out]
            n256 = invoke class="VI" method="FP.Open"(reference=w435, error in=w436, "Activate"=TRUE ("Activate?"), "State"=T7."Standard") -> ()  [unwired: 1 in, 5 out]
          }
          frame "TE Complete" {
            w439 = FALSE ("Blinking")
            w440 = T1."Completed" ("Test State")
            # "Message From TE"
            n257 = invoke on="Nest" class="Str" method="Reinit To Default"() -> ()  [unwired: 3 in, 3 out]
            n258 = property on="Test Running" class="Bool (strict)"("Blinking"=w439, "Value"=w439) -> ()  [unwired: 2 in, 2 out]
            n259 = invoke on="SN" class="Str" method="Reinit To Default"() -> ()  [unwired: 3 in, 3 out]
            n260 = call <vilib>:"Q.Enqueue Task.vi"("Task Name"="PLC - Set Done", "Q In"=w438) -> ()  [unwired: 8 in, 2 out]
            n261 = Bundle By Name(cluster=w442, "State"=w440) -> (w441:T8)
            n262 = local write "Test State"(w440) -> ()
          }
          frame "TE Enable PLC" {
            n263 = Variant To Data(type=FALSE, Variant=w446) -> (data=w444:bool)  [unwired: 1 in, 1 out]
            n264 = local write "Enabled"(w444) -> ()
          }
          frame "TE Idle" {
            # "Message From TE"
          }
          frame "TE PLC Start" {
            n265 = call <vilib>:"Q.Enqueue Task.vi"("Task Name"="PLC - Set Start", "Q In"=w450) -> ()  [unwired: 8 in, 2 out]
          }
          frame "TE Launch" {
            # "Message to TE"
            n266 = case shown="True" w452 {
              tunnel: w453 -> [_ w467]
              tunnel: [_ w464] -> _
              frame False {
              }
              frame True {
                n267 = local read "Nest"() -> (w456:string)
                n268 = local read "SN"() -> (w455:string)
                n269 = call <vilib>:"Q.Enqueue Seq.vi"("Seq Task Name"="Test Reset" ("Task Name"), "Q In"=w467) -> ("Q Out"=w458:refnum<queue>)  [unwired: 8 in, 1 out]
                n270 = To Variant(anything=w455) -> (Variant=w463:variant)
                n271 = call <vilib>:"Q.Enqueue Task.vi"("Data1"=w463, "Task Name"="Set SN", "Q In"=w458) -> ("Q Out"=w459:refnum<queue>)  [unwired: 7 in, 1 out]
                n272 = To Variant(anything=w456) -> (Variant=w461:variant)
                n273 = call <vilib>:"Q.Enqueue Task.vi"("Data1"=w461, "Task Name"="Set UUT Pos", "Q In"=w459) -> ("Q Out"=w457:refnum<queue>)  [unwired: 7 in, 1 out]
                n274 = call <vilib>:"Q.Enqueue Seq.vi"("Seq Task Name"="Test Start", "Q In"=w457) -> ("error out"=w464:errorcluster)  [unwired: 8 in, 1 out]
              }
            }
          }
          frame "TE Result" {
            # "Message From TE"
            n275 = Variant To Data(type="", Variant=w472) -> (data=→"Result":string)  [unwired: 1 in, 1 out]
            n276 = call <vilib>:"Q.Enqueue Task.vi"("Task Name"="PLC - Set Result", "Q In"=w469) -> ()  [unwired: 8 in, 2 out]
          }
          frame "TE Running" {
            # "Message From TE"
            n277 = call <vilib>:"Q.Enqueue Task.vi"("Task Name"="PLC - Clear Ready", "Q In"=w475) -> ()  [unwired: 8 in, 2 out]
            n278 = property on="Test Running" class="Bool (strict)"("Blinking"=TRUE) -> ()  [unwired: 2 in, 2 out]
            "Test Running" <- TRUE ("Test Running")
          }
          frame Default {
          }
        }
      }
      frame "Error", Default {
        n279 = case shown="Default" w485 {
          tunnel: w484 -> [_ w489 _]
          tunnel: [w486 w489 _] -> w483
          tunnel: w482 -> [w488 _ _]
          frame "Error" {
            n280 = Variant To Data(type=errorcluster {"status"=FALSE, "code"=0, "source"=""} ("error constant"), Variant=w488) -> (data=w486:errorcluster)  [unwired: 1 in, 1 out]
          }
          frame Default {
          }
          frame "Clear" {
          }
        }
        "Error" <- w483
        n281 = Get Date/Time In Seconds() -> (seconds since 1Jan1904=→"Error Time":timestamp)
      }
      frame "Exit" {
        n282 = Generate User Event(user event=w494, event data cluster=TRUE ("event data")) -> ()  [unwired: 2 in, 2 out]
        n283 = case shown="False" w492 {
          frame False {
            n284 = call <vilib>:"Scheduler.Exit.vi"() -> ()  [unwired: 11 in, 1 out]
          }
          frame True {
          }
        }
        n285 = control-ref of="This VI"() -> (w491:refnum<vi>)
        n286 = property class="VI"(reference=w491, "FP.State"=T7."Closed" ("Front Panel Window:State")) -> ()  [unwired: 1 in, 2 out]
      }
    }
  }
